vi "Serial Read.vi"(8 "error in (no error)":errorcluster, 11 "VISA resource name in":refnum<visa-resource-name>) -> (0 "error out":errorcluster, 2 "Serial Response":string, 3 "VISA resource name out":refnum<visa-resource-name>)   [LabVIEW 2020, in "Serial device.lvclass"]
doc: "SubVI para facilitar la realización de leer la respuesta del micro"
uses:
  Serial device.lvclass
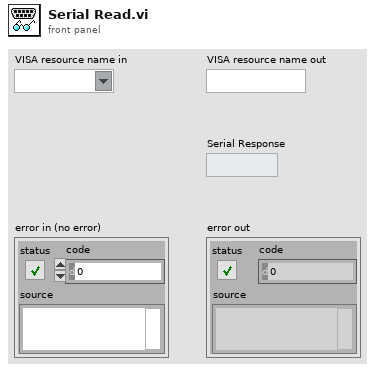
[diagram p1: front panel]
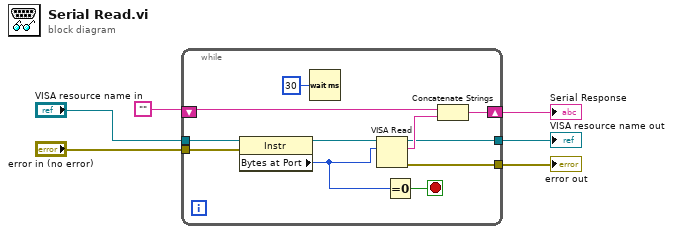
[diagram p0: block diagram]
diagram:
  n1 = while {
    tunnel: "VISA resource name in" -> [w17]
    tunnel: "error in (no error)" -> [w16]
    tunnel: [w12] -> w4
    shift-right: [w11] -> w3
    shift-left: "" -> [w10]
    tunnel: [w8] -> w2
    stop <- w13 stop-if-true
    n2 = property class="Instr"(reference=w17, error in=w16) -> (reference out=w15:refnum<visa-resource-name>, "Bytes at Port"=w14:u32)  [unwired: 1 out]
    n3 = Wait (ms)(milliseconds to wait=u32 30) -> ()  [unwired: 1 out]
    n4 = VISA Read(VISA resource name=w15, byte count=w14) -> (VISA resource name out=w8:refnum<visa-resource-name>, read buffer=w9:string, error out=w12:errorcluster)  [unwired: 1 in, 1 out]
    n5 = Equal To 0?(x=w14) -> (x = 0?=w13:bool)
    n6 = Concatenate Strings(w10, w9) -> (w11:string)
  }
  "error out" <- w4
  "VISA resource name out" <- w2
  "Serial Response" <- w3
